vi "Explore_Open.vi"(7 "JPG":refnum<vi>, 8 "Task":enum16{"run", "open"}(ring), 9 "queueName":string="PV_script", 10 "Name":string, 11 "String in":refnum<vi>) -> ()   [LabVIEW 2022 SP3]
panel:
  out "JPG":picture
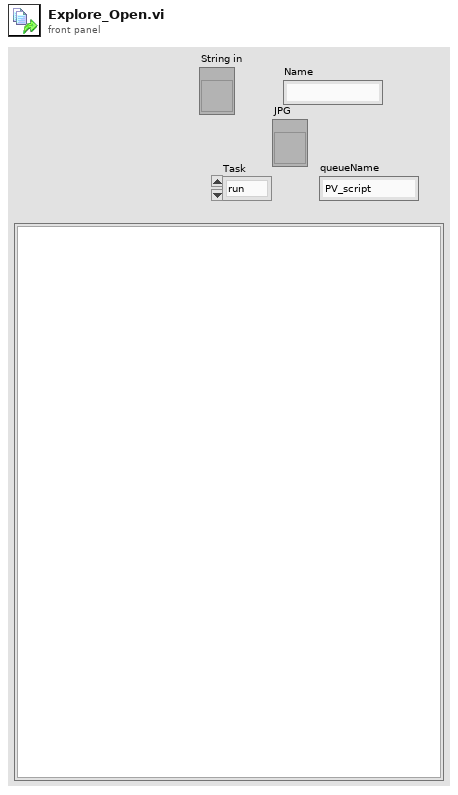
[diagram p1: front panel]
types:
  T1 = enum32{"Invalid", "Standard", "Closed", "Hidden", "Minimized", "Maximized"}
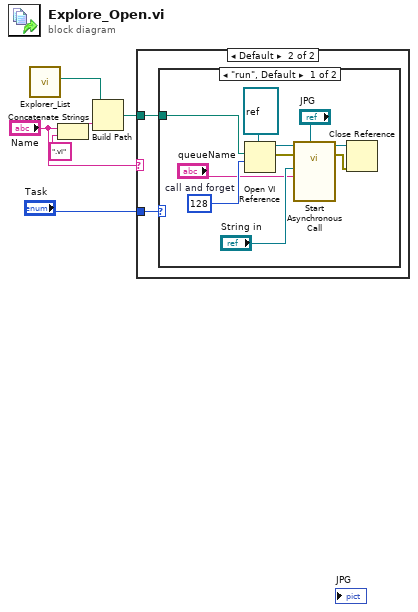
[diagram p0: block diagram]
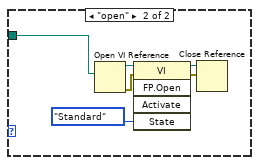
[diagram p3: hidden frame]
diagram:
  n1 = call "Explorer_List.vi"() -> ("Explore Path"=w6:path)  [unwired: 9 in, 2 out]
  n2 = Concatenate Strings("Name", ".vi" ("string")) -> (w2:string)
  n3 = Build Path(base path=w6, name or relative path=w2) -> (appended path=w5:path)
  n4 = case shown="Default" "Name" {
    tunnel: w5 -> [_ w8]
    tunnel: "Task" -> [_ w7]
    frame "" {
    }
    frame Default {
      n5 = case shown="\"run\", Default" w7 {
        tunnel: w8 -> [w11 w24]
        frame "run", Default {
          w17 = 128  # call and forget
          n6 = Open VI Reference(type specifier VI Refnum (for type only)=refnum<vi> refnum, vi path=w11, options=w17) -> (vi reference=w12:refnum<vi>, error out=w15:errorcluster)  [unwired: 3 in]
          n7 = call-by-ref "Start Asynchronous Call"(reference=w12, error in=w15, "JPG"="JPG", "queueName"="queueName", "Console Reference"="String in") -> (reference out=w14:refnum<vi>, error out=w13:errorcluster)  [unwired: 9 in]
          n8 = Close Reference(reference=w14, error in (no error)=w13) -> ()  [unwired: 1 out]
        }
        frame "open" {
          n9 = Open VI Reference(vi path=w24) -> (vi reference=w23:refnum<vi>, error out=w22:errorcluster)  [unwired: 5 in]
          n10 = invoke class="VI" method="FP.Open"(reference=w23, error in=w22, "State"=T1."Standard") -> (reference out=w21:refnum<vi>, error out=w20:errorcluster)  [unwired: 2 in, 3 out]
          n11 = Close Reference(reference=w21, error in (no error)=w20) -> ()  [unwired: 1 out]
        }
      }
    }
  }
